vi "Read channels.vi"(8 "error in (no error)":errorcluster, 11 "Parallel Step Config in":refnum<class "Parallel Step Config.lvclass">) -> (0 "error out":errorcluster, 2 "Channels":refnum<class "TBM channel.lvclass">[](array[class]), 3 "Parallel Step Config out":refnum<class "Parallel Step Config.lvclass">)   [LabVIEW 2015, in "Parallel Step Config.lvclass"]
uses:
  Parallel Step Config.lvclass
  <vilib>/NI/Tag Bus Module Framework/channel/TBM channel.lvclass
  Parallel Step Config.lvclass/Parallel Step Config.ctl
  <vilib>/NI/Tag Bus/tag/tag descriptor.lvclass/tag descriptor.ctl
  <vilib>/NI/Tag Bus/tag/read tag name.vi
  classes/Step/Config/Step Config.lvclass
  <vilib>/NI/Tag Bus/tag/tag descriptor.lvclass
panel:
  out "Array":i32[](array[numeric])
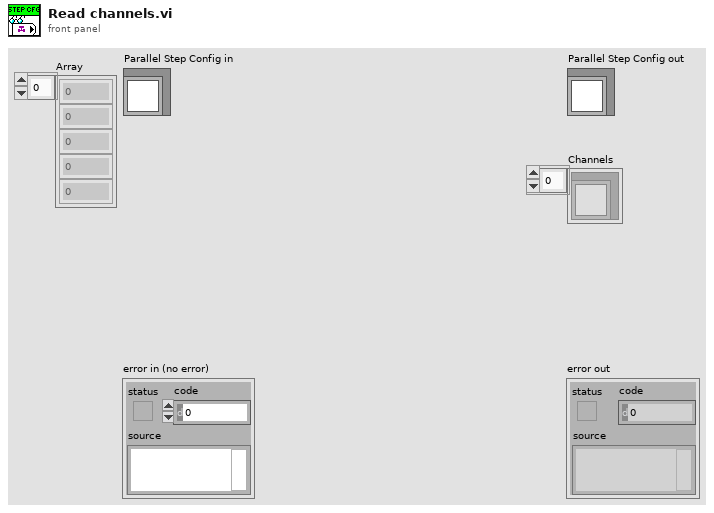
[diagram p1: front panel]
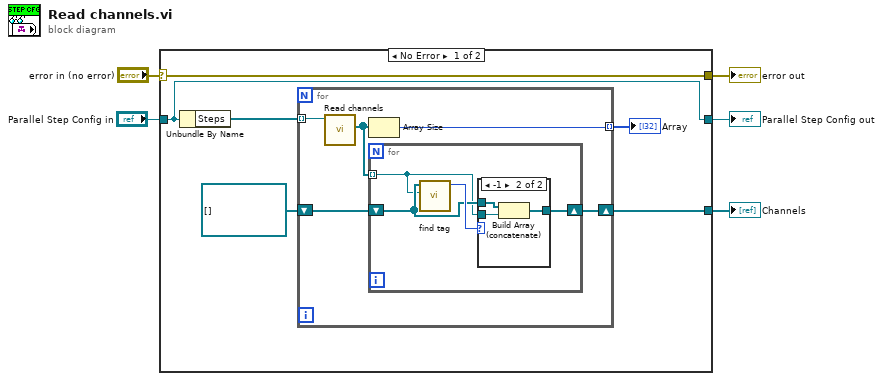
[diagram p0: block diagram]
diagram:
  n1 = case shown="No Error" "error in (no error)" {
    selector: "error in (no error)" -> [w11 w26]
    tunnel: [w11 w26] -> w2
    tunnel: [w10 w25] -> w4
    tunnel: "Parallel Step Config in" -> [w10 w25]
    tunnel: [w7 _] -> w1
    frame No Error {
      n2 = Unbundle By Name(w10) -> ("Steps"=w9:refnum<class "Step Config.lvclass">[])
      n3 = for {
        tunnel: w9 -> [w16] mode=indexing
        shift-right: [w14] -> w7
        shift-left: refnum<class "TBM channel.lvclass">[] [] ("Channels") -> [w15]
        tunnel: [w12] -> w6 mode=indexing
        n4 = call-dynamic "Read channels.vi"("Step Config in"=w16) -> ("Channels"=w13:refnum<class "TBM channel.lvclass">[])  [unwired: 8 in, 2 out]
        n5 = Array Size(array=w13) -> (size(s)=w12:i32)
        n6 = for {
          tunnel: w13 -> [w17] mode=indexing
          shift-right: [w19] -> w14
          shift-left: w15 -> [w18]
          n7 = call <vilib>:"find tag.vi"("tag"=w17, "tags in"=w18) -> ("index"=w20:i32)  [unwired: 9 in]
          n8 = case shown="-1" w20 {
            tunnel: [w21 w22] -> w19
            tunnel: w18 -> [w21 w24]
            tunnel: w17 -> [_ w23]
            frame 0, Default {
            }
            frame -1 {
              n9 = Build Array (concatenate)(w24, w23) -> (w22:refnum<class "TBM channel.lvclass">[])
            }
          }
        }
      }
      "Array" <- w6
    }
    frame Error {
    }
  }
  "error out" <- w2
  "Parallel Step Config out" <- w4
  "Channels" <- w1
